vi "Self-test_example.vi"() -> ()   [LabVIEW 2017, in "labview-standard-library.lvlib"]
uses:
  labview-standard-library.lvlib
  universial-controls/Driver_inputs.ctl
panel:
  out "x*y 2":dbl
  out "x*y":dbl
  in  "stop":bool
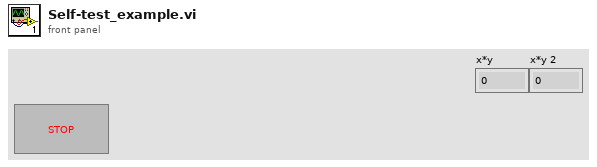
[diagram p1: front panel]
types:
  T1 = typedef "labview-standard-library.lvlib/Driver_inputs.ctl" = cluster{"current time":timestamp, "Left Joy":dbl, "Right Joy":dbl, "Self-test?":bool}
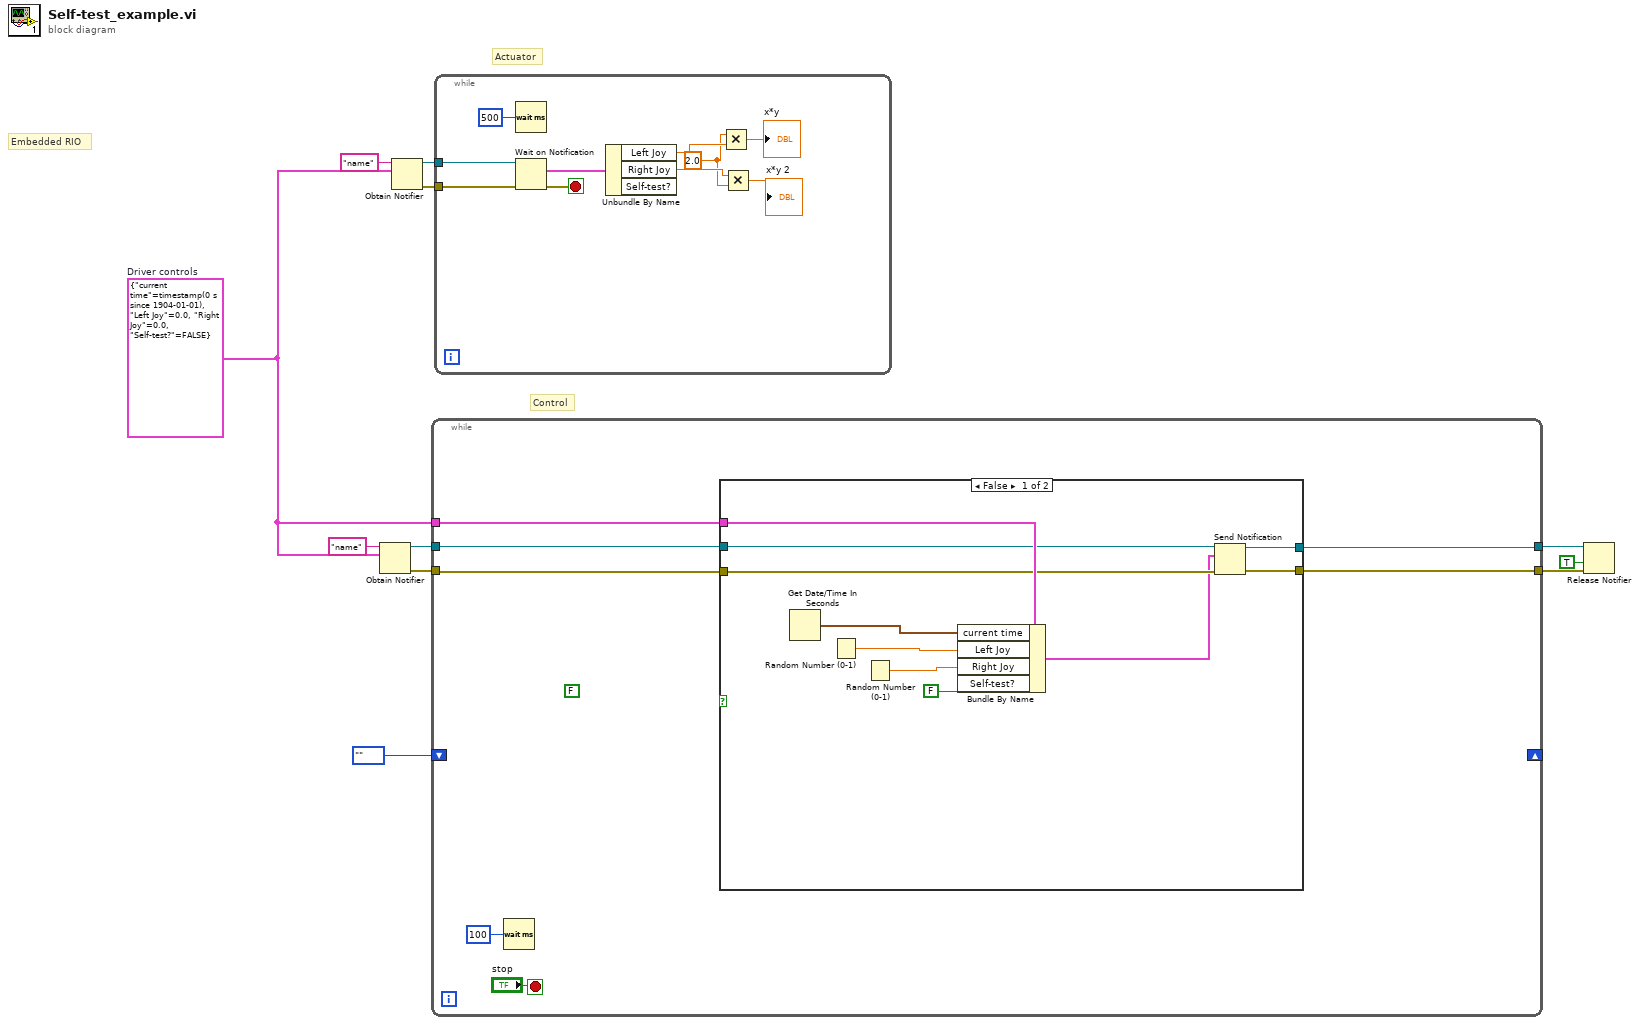
[diagram p0: block diagram]
diagram:
  w2 = T1 {"current time"=timestamp(0 s since 1904-01-01), "Left Joy"=0.0, "Right Joy"=0.0, "Self-test?"=FALSE}  # Driver controls
  # "Embedded RIO"
  # "Control"
  # "Actuator"
  n1 = Obtain Notifier(name (unnamed)="name", notification data type=w2) -> (notifier out=w11:refnum<notifier>, error out=w10:errorcluster)  [unwired: 2 in, 1 out]
  n2 = Obtain Notifier(name (unnamed)="name", notification data type=w2) -> (notifier out=w4:refnum<notifier>, error out=w3:errorcluster)  [unwired: 2 in, 1 out]
  n3 = while {
    tunnel: w11 -> [w13]
    tunnel: w10 -> [w12]
    tunnel: [w15] -> w8
    tunnel: [w14] -> w7
    tunnel: w2 -> [w16]
    shift-right: _ -> [_]
    shift-left: enum16{""}."" -> [_]
    stop <- "stop" stop-if-true
    (unwired) FALSE
    n4 = Wait (ms)(milliseconds to wait=u32 100) -> ()  [unwired: 1 out]
    n5 = case shown="False" {
      selector: _ -> [_ _]
      tunnel: w16 -> [w27 _]
      tunnel: [w26 _] -> w15
      tunnel: [w25 _] -> w14
      tunnel: w13 -> [w24 _]
      tunnel: w12 -> [w23 _]
      frame False {
        n6 = Get Date/Time In Seconds() -> (seconds since 1Jan1904=w19:timestamp)
        n7 = Random Number (0-1)() -> (number: 0 to 1=w20:dbl)
        n8 = Random Number (0-1)() -> (number: 0 to 1=w21:dbl)
        n9 = Bundle By Name(cluster=w27, "current time"=w19, "Left Joy"=w20, "Right Joy"=w21, "Self-test?"=FALSE) -> (w22:T1)
        n10 = Send Notification(notification=w22, notifier=w24, error in (no error)=w23) -> (notifier out=w26:refnum<notifier>, error out=w25:errorcluster)
      }
      frame True {
      }
    }
  }
  n11 = while {
    tunnel: w4 -> [w37]
    tunnel: w3 -> [w36]
    stop <- w35 stop-if-true
    w31 = 2.0
    n12 = Wait (ms)(milliseconds to wait=u32 500) -> ()  [unwired: 1 out]
    n13 = Wait on Notification(notifier=w37, error in (no error)=w36) -> (notification=w34:T1, error out=w35:errorcluster)  [unwired: 2 in, 2 out]
    n14 = Unbundle By Name(w34) -> ("Left Joy"=w33:dbl, "Right Joy"=w32:dbl)  [unwired: 1 out]
    n15 = Multiply(x=w31, y=w33) -> (x*y=→"x*y":dbl)
    n16 = Multiply(x=w32, y=w31) -> (x*y=→"x*y 2":dbl)
  }
  n17 = Release Notifier(notifier=w8, force destroy? (F)=TRUE, error in (no error)=w7) -> ()  [unwired: 3 out]
